vi "Temperhum.ThorOpen.vi"() -> ()   [LabVIEW 2019, in "TEMPerHUM.lvlib"]
uses:
  SMOs/TEMPerHUM/TEMPerHUM.lvlib
panel:
  out "instrument handle out":refnum<visa-resource-name>
  out "Computer Name":string
  out "error out":errorcluster
  in  "error in (no error)":errorcluster
  out "Device Handle":i64
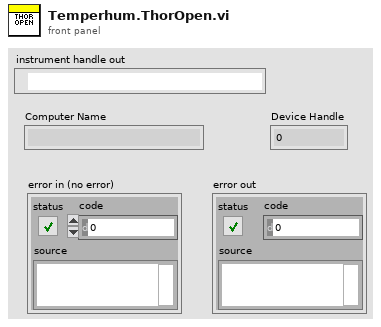
[diagram p1: front panel]
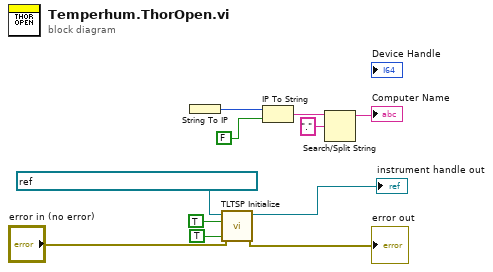
[diagram p0: block diagram]
diagram:
  n1 = String To IP() -> (0:w11:u32)  [unwired: 1 in]
  n2 = call <instrlib>:"TLTSP Initialize.vi"("error in (no error)"="error in (no error)", "Reset Device (Reset Device)"=TRUE, "ID Query (Do Query)"=TRUE, "resource name"=refnum<visa-resource-name> "USB0::0x1313::0x80F8::M00410498::INSTR") -> ("error out"=→"error out":errorcluster, "instrument handle out"=→"instrument handle out":refnum<visa-resource-name>)  [unwired: 6 in]
  n3 = IP To String(1:FALSE, 2:w11) -> (0:w7:string)
  n4 = Search/Split String(string=w7, search string/char (-)=".") -> (substring before match=→"Computer Name":string)  [unwired: 1 in, 2 out]
